vi "编程口协议.vi"(11 "串口号":refnum<visa-resource-name>="COM2") -> (0 "错误输出":errorcluster, 3 "VISA资源名称输出":refnum<visa-resource-name>)   [LabVIEW 2014]
panel:
  out "X17":bool
  out "X16":bool
  out "D0":i32
  out "D1":i32
  out "D2":i32
  out "D3":i32
  out "D7":i32
  out "D6":i32
  out "D5":i32
  out "D4":i32
  out "D9":i32
  out "D8":i32
  out "Y37":bool
  out "Y36":bool
  out "Y35":bool
  out "Y34":bool
  out "Y33":bool
  out "Y32":bool
  out "Y31":bool
  out "Y30":bool
  out "Y27":bool
  out "Y26":bool
  out "Y25":bool
  out "Y24":bool
  out "Y23":bool
  out "Y22":bool
  out "Y21":bool
  out "Y20":bool
  out "Y17":bool
  out "Y16":bool
  out "Y15":bool
  out "Y14":bool
  out "Y13":bool
  out "Y12":bool
  out "Y11":bool
  out "Y10":bool
  out "Y7":bool
  out "Y6":bool
  out "Y5":bool
  out "Y4":bool
  out "Y3":bool
  out "Y2":bool
  out "Y1":bool
  out "Y0":bool
  out "M31":bool
  out "M30":bool
  out "M29":bool
  out "M28":bool
  out "M27":bool
  out "M26":bool
  out "M25":bool
  out "M24":bool
  out "M23":bool
  out "M22":bool
  out "?":bool
  out "M20":bool
  out "M19":bool
  out "M18":bool
  out "M17":bool
  out "M16":bool
  out "M15":bool
  out "M14":bool
  out "M13":bool
  out "M12":bool
  out "M11":bool
  out "M10":bool
  out "M9":bool
  out "M8":bool
  out "M7":bool
  out "M6":bool
  out "M5":bool
  out "M4":bool
  out "M3":bool
  out "M2":bool
  out "M1":bool
  out "M0":bool
  out "X37":bool
  out "X36":bool
  out "X35":bool
  out "X34":bool
  out "X33":bool
  out "X32":bool
  out "X31":bool
  out "X30":bool
  out "X27":bool
  out "X26":bool
  out "X25":bool
  out "X24":bool
  out "X23":bool
  out "X22":bool
  out "X21":bool
  out "X20":bool
  out "X15":bool
  out "X14":bool
  out "X13":bool
  out "X12":bool
  out "X11":bool
  out "X10":bool
  out "X7":bool
  out "X6":bool
  out "X5":bool
  out "X4":bool
  out "X3":bool
  out "X2":bool
  out "X1":bool
  out "X0":bool
  in  "停止":bool
  # "三菱F3GA系列PLC  I/O监视"
  # "读Y0-Y7"
  # "读X0-X7"
  # "读M0-M7"
  # "读Y10-Y17"
  # "读M8-M15"
  # "读X10-X17"
  # "读Y20-Y27"
  # "读M16-M23"
  # "读X20-X27"
  # "读M24-M31"
  # "读Y30-Y37"
  # "读X30-X37"
  # "读D0-D4"
  # "读D5-D9"
  # "确保程序运行正常 设置好串口号 . 波特率.  然后再启动程序"
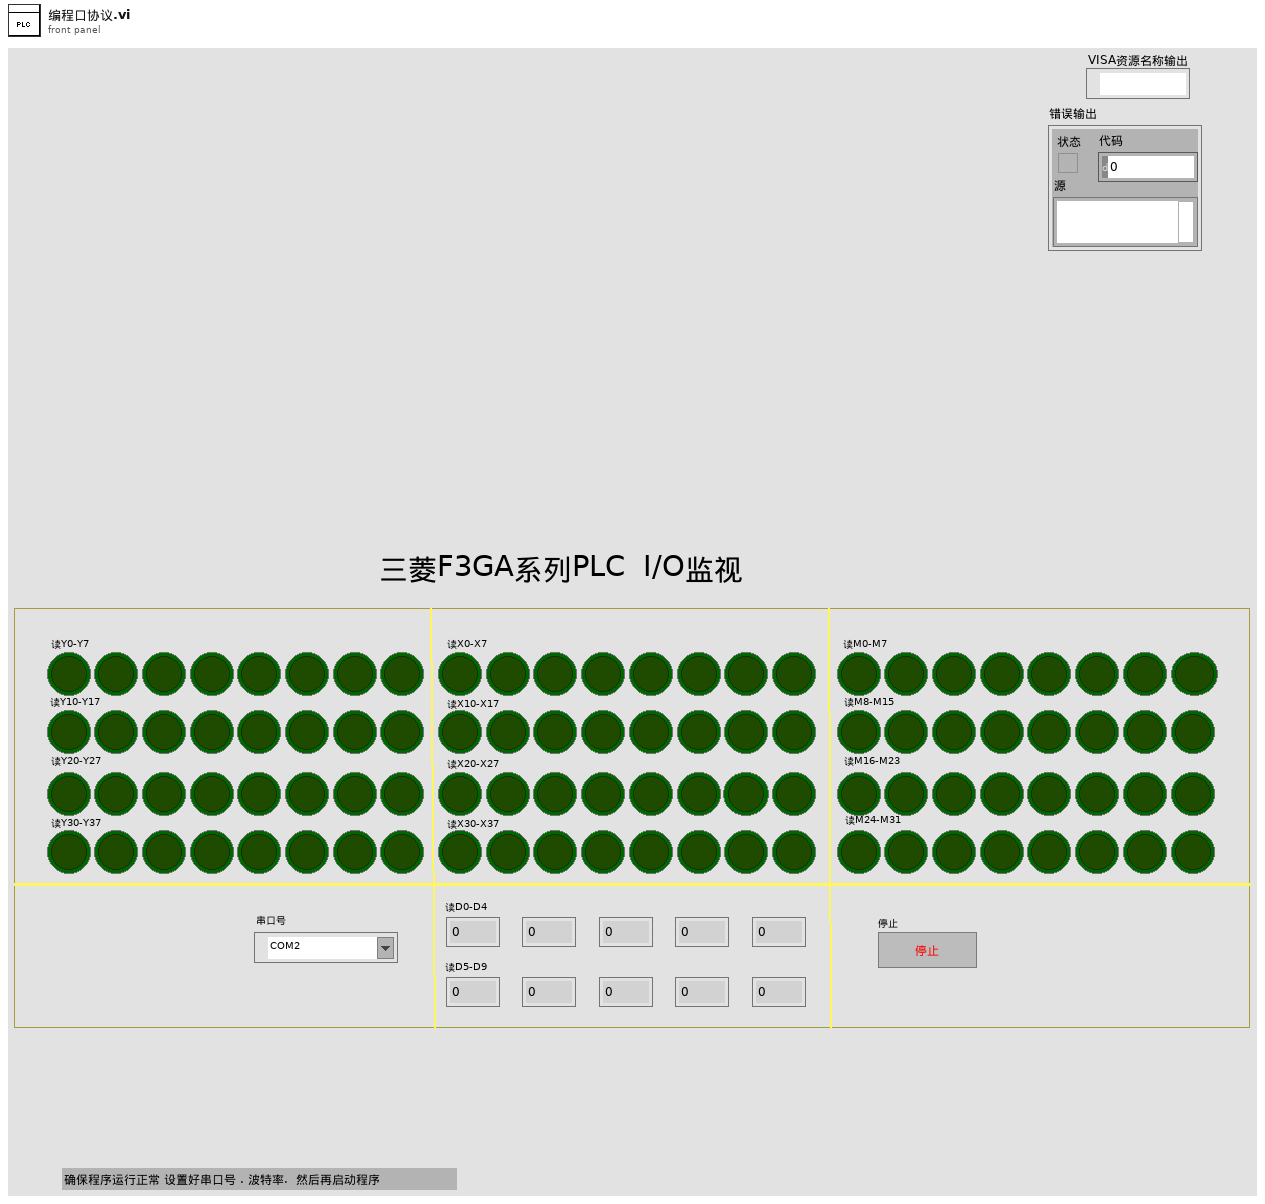
[diagram p1: front panel]
types:
  T1 = cluster{"X0":bool, "X1":bool, "X2":bool, "X3":bool, "X4":bool, "X5":bool, "X6":bool, "X7":bool, "X10":bool, "X11":bool, "X12":bool, "X13":bool, "X14":bool, "X15":bool, "X16":bool, "X17":bool}
  T2 = cluster{"X20":bool, "X21":bool, "X22":bool, "X23":bool, "X24":bool, "X25":bool, "X26":bool, "X27":bool, "X30":bool, "X31":bool, "X32":bool, "X33":bool, "X34":bool, "X35":bool, "X36":bool, "X37":bool}
  T3 = cluster{"M16":bool, "M17":bool, "M18":bool, "M19":bool, "M20":bool, "M21":bool, "M22":bool, "M23":bool, "M24":bool, "M25":bool, "M26":bool, "M27":bool, "M28":bool, "M29":bool, "M30":bool, "M31":bool}
  T4 = cluster{"M0":bool, "M1":bool, "M2":bool, "M3":bool, "M4":bool, "M5":bool, "M6":bool, "M7":bool, "M8":bool, "M9":bool, "M10":bool, "M11":bool, "M12":bool, "M13":bool, "M14":bool, "M15":bool}
  T5 = cluster{"Y0":bool, "Y1":bool, "Y2":bool, "Y3":bool, "Y4":bool, "Y5":bool, "Y6":bool, "Y7":bool, "Y10":bool, "Y11":bool, "Y12":bool, "Y13":bool, "Y14":bool, "Y15":bool, "Y16":bool, "Y17":bool}
  T6 = cluster{"Y20":bool, "Y21":bool, "Y22":bool, "Y23":bool, "Y24":bool, "Y25":bool, "Y26":bool, "Y27":bool, "Y30":bool, "Y31":bool, "Y32":bool, "Y33":bool, "Y34":bool, "Y35":bool, "Y36":bool, "Y37":bool}
  T7 = cluster{"D0":i32, "D1":i32, "D2":i32, "D3":i32, "D4":i32, "D5":i32, "D6":i32, "D7":i32, "D8":i32, "D9":i32}
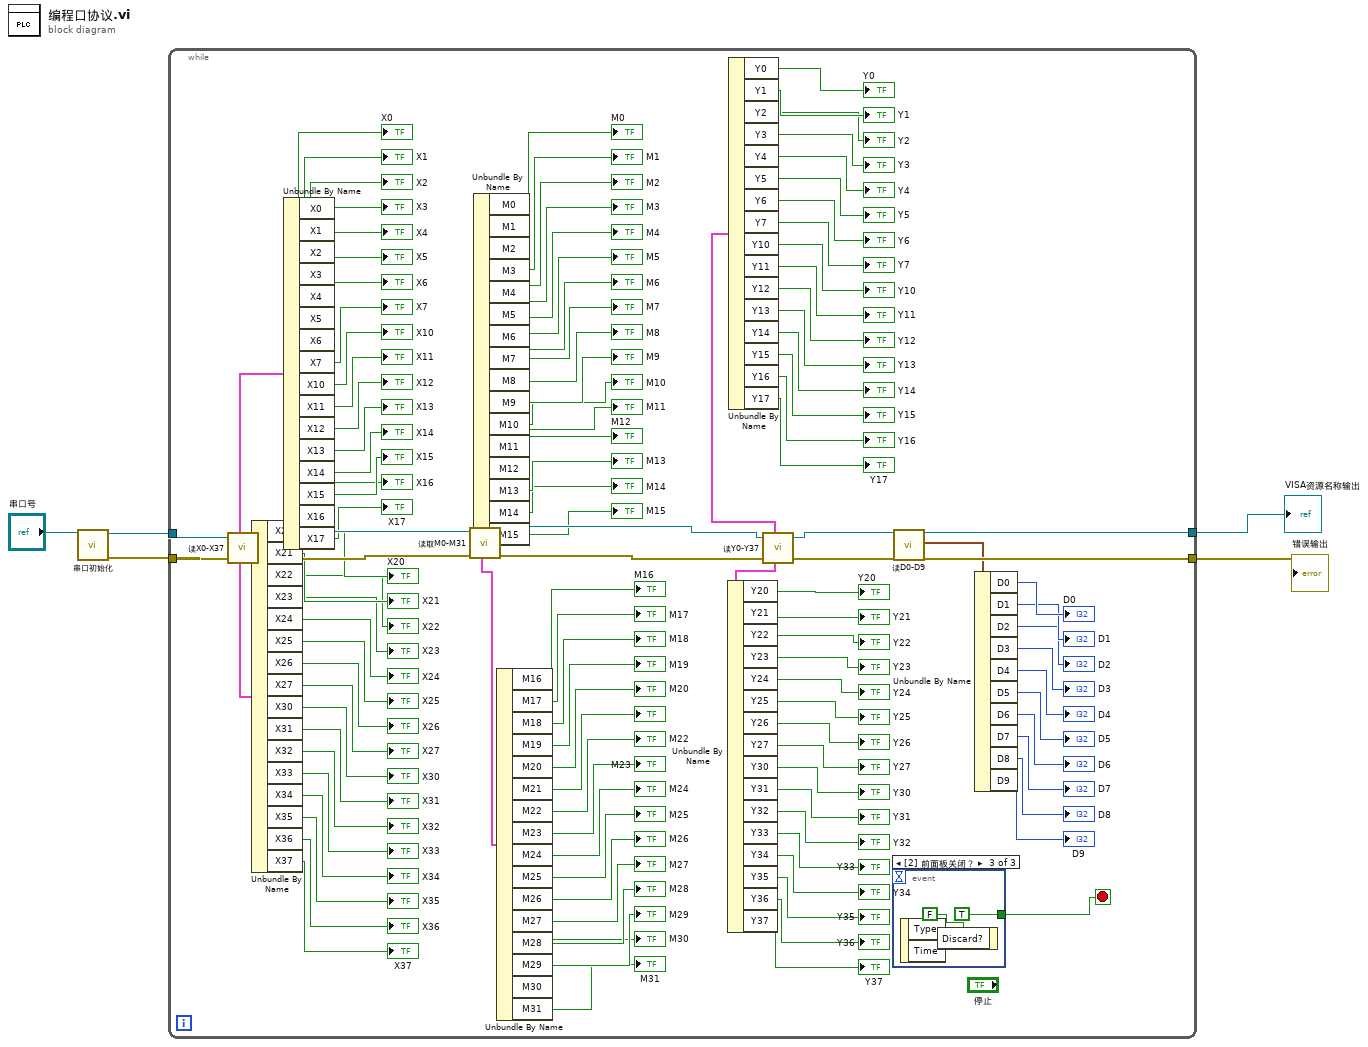
[diagram p0: block diagram]
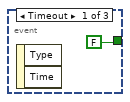
[diagram p2: hidden frame]
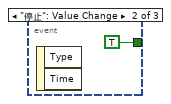
[diagram p3: hidden frame]
diagram:
  n1 = call "串口初始化.vi"("VISA引用句柄输入"="串口号") -> ("错误输出"=w4:errorcluster, "VISA引用句柄输出"=w5:refnum<visa-resource-name>)  [unwired: 9 in]
  n2 = while {
    tunnel: w5 -> [w129]
    tunnel: w4 -> [w128]
    tunnel: [w19] -> w2
    tunnel: [w18] -> w1
    stop <- w6 stop-if-true
    n3 = call "读X0-X37.vi"("VISA资源名称"=w129, "错误输入（无错误）"=w128) -> ("X0-X17"=w121:T1, "X20-X37"=w120:T2, "VISA资源名称输出"=w127:refnum<visa-resource-name>, "错误输出"=w126:errorcluster)  [unwired: 4 in]
    n4 = Unbundle By Name(w120) -> ("X20"=→"X20":bool, "X21"=→"X21":bool, "X22"=→"X22":bool, "X23"=→"X23":bool, "X24"=→"X24":bool, "X25"=→"X25":bool, "X26"=→"X26":bool, "X27"=→"X27":bool, "X30"=→"X30":bool, "X31"=→"X31":bool, "X32"=→"X32":bool, "X33"=→"X33":bool, "X34"=→"X34":bool, "X35"=→"X35":bool, "X36"=→"X36":bool, "X37"=→"X37":bool)
    n5 = Unbundle By Name(w121) -> ("X0"=→"X0":bool, "X1"=→"X1":bool, "X2"=→"X2":bool, "X3"=→"X3":bool, "X4"=→"X4":bool, "X5"=→"X5":bool, "X6"=→"X6":bool, "X7"=→"X7":bool, "X10"=→"X10":bool, "X11"=→"X11":bool, "X12"=→"X12":bool, "X13"=→"X13":bool, "X14"=→"X14":bool, "X15"=→"X15":bool, "X16"=→"X16":bool, "X17"=→"X17":bool)
    n6 = call "读取M0-M31.vi"("错误输入（无错误）"=w126, "VISA资源名称"=w127) -> ("错误输出"=w124:errorcluster, "VISA资源名称输出"=w125:refnum<visa-resource-name>, "M16-M21"=w88:T3, "M0-M15"=w89:T4)  [unwired: 6 in]
    n7 = Unbundle By Name(w89) -> ("M0"=→"M0":bool, "M1"=→"M1":bool, "M2"=→"M2":bool, "M3"=→"M3":bool, "M4"=→"M4":bool, "M5"=→"M5":bool, "M6"=→"M6":bool, "M7"=→"M7":bool, "M8"=→"M8":bool, "M9"=→"M9":bool, "M10"=→"M10":bool, "M11"=→"M11":bool, "M12"=→"M12":bool, "M13"=→"M13":bool, "M14"=→"M14":bool, "M15"=→"M15":bool)
    n8 = Unbundle By Name(w88) -> ("M16"=→"M16":bool, "M17"=→"M17":bool, "M18"=→"M18":bool, "M19"=→"M19":bool, "M20"=→"M20":bool, "M21"=→"?":bool, "M22"=→"M22":bool, "M23"=→"M23":bool, "M24"=→"M24":bool, "M25"=→"M25":bool, "M26"=→"M26":bool, "M27"=→"M27":bool, "M28"=→"M28":bool, "M29"=→"M29":bool, "M30"=→"M30":bool, "M31"=→"M31":bool)
    n9 = call "读Y0-Y37.vi"("VISA资源名称"=w125, "错误输入（无错误）"=w124) -> ("Y0-Y17"=w55:T5, "Y20-Y37"=w54:T6, "VISA资源名称输出"=w123:refnum<visa-resource-name>, "错误输出"=w122:errorcluster)  [unwired: 4 in]
    n10 = Unbundle By Name(w54) -> ("Y20"=→"Y20":bool, "Y21"=→"Y21":bool, "Y22"=→"Y22":bool, "Y23"=→"Y23":bool, "Y24"=→"Y24":bool, "Y25"=→"Y25":bool, "Y26"=→"Y26":bool, "Y27"=→"Y27":bool, "Y30"=→"Y30":bool, "Y31"=→"Y31":bool, "Y32"=→"Y32":bool, "Y33"=→"Y33":bool, "Y34"=→"Y34":bool, "Y35"=→"Y35":bool, "Y36"=→"Y36":bool, "Y37"=→"Y37":bool)
    n11 = Unbundle By Name(w55) -> ("Y0"=→"Y0":bool, "Y1"=→"Y1":bool, "Y2"=→"Y2":bool, "Y3"=→"Y3":bool, "Y4"=→"Y4":bool, "Y5"=→"Y5":bool, "Y6"=→"Y6":bool, "Y7"=→"Y7":bool, "Y10"=→"Y10":bool, "Y11"=→"Y11":bool, "Y12"=→"Y12":bool, "Y13"=→"Y13":bool, "Y14"=→"Y14":bool, "Y15"=→"Y15":bool, "Y16"=→"Y16":bool, "Y17"=→"Y17":bool)
    n12 = event shown="[2] 前面板关闭？" {
      selector: _ -> [_ _ _]
      dyn-events: _ -> [_ _ _]
      timeout: _ -> [_ _ _]
      tunnel: [FALSE TRUE TRUE] -> w6
      event Timeout {
        n13 = event-data() -> ()  [unwired: 1 in, 2 out]
      }
      event "停止": Value Change {
        n14 = event-data() -> ()  [unwired: 1 in, 2 out]
      }
      event Panel Close? {
        n15 = event-data() -> ()  [unwired: 1 in, 2 out]
        n16 = event-data("Discard?"=FALSE ("放弃？")) -> ()  [unwired: 1 in, 1 out]
      }
    }
    n17 = call "读D0-D9.vi"("VISA资源名称"=w123, "错误输入（无错误）"=w122) -> ("VISA资源名称输出"=w19:refnum<visa-resource-name>, "D0-D9"=w17:T7, "错误输出"=w18:errorcluster)  [unwired: 15 in]
    n18 = Unbundle By Name(w17) -> ("D0"=→"D0":i32, "D1"=→"D1":i32, "D2"=→"D2":i32, "D3"=→"D3":i32, "D4"=→"D4":i32, "D5"=→"D5":i32, "D6"=→"D6":i32, "D7"=→"D7":i32, "D8"=→"D8":i32, "D9"=→"D9":i32)
  }
  "VISA资源名称输出" <- w2
  "错误输出" <- w1
